vi "AlliGator Compute Shot Noise Average Lifetime Simulation Histograms.vi"(0 "Average Lifetimes (Pure Poisson)":dbl[](array[numeric]), 1 "Histogram Bin Size":dbl[unit], 5 "Average Lifetimes (AlliGator)":dbl[](array[numeric]), 7 "Lifetime Histo Percentiles":dbl[](array[numeric])=[99.0, 1.0], 9 "Average Lifetime SDVs (AlliGator)":dbl[](array[numeric]), 11 "Error In":errorcluster, 12 "Histogram Bin Size (SDV)":dbl[unit], 13 "SDV Histo Percentiles":dbl[](array[numeric])=[99.0, 1.0]) -> (3 "Histograms":cluster{"Axis":dbl[], "Histogram":dbl[]}[](array[cluster]), 4 "Array Statistic (Pure Poisson)":T1, 6 "Array Statistics (AlliGator)":T1, 10 "Array Statistics (AlliGator SDVs)":T1, 14 "Message":string, 15 "Error Out":errorcluster)   [LabVIEW 2021, in "AlliGator Shot Noise Influence on Average Lifetime.lvlib"]
doc: "Computes histograms and summary statistics for the computed lifetimes."
uses:
  AlliGator Shot Noise Influence on Average Lifetime.lvlib
  Arrays/Array Statistics.ctl
  Histograms/Linear Histogram Options.ctl
  Histograms/Histogram Bin Option.ctl
  Histograms/Histogram Bin Position.ctl
  5e0c3266-499e-46b2-80ef-c194e49f915b.vi
  9765538f-b151-4b8e-9b71-29b00fbc2fe4.vi
  8faa86fc-1a47-49e1-a18e-559db2184d30.vi
  c2a6bf4c-2b36-4ed5-885f-cf0e0406484b.vi
  6ac06ea2-d37e-43e0-baed-35fadc42c3ab.vi
  6045f332-e983-43bb-9ace-d0f5cff48457.vi
  5e0c3266-499e-46b2-80ef-c194e49f915b.vi/1ce800e1-bcd7-4855-83e2-66cab3687e54.vi
  9765538f-b151-4b8e-9b71-29b00fbc2fe4.vi/1ce800e1-bcd7-4855-83e2-66cab3687e54.vi
  8faa86fc-1a47-49e1-a18e-559db2184d30.vi/1ce800e1-bcd7-4855-83e2-66cab3687e54.vi
  c2a6bf4c-2b36-4ed5-885f-cf0e0406484b.vi/e021cd17-e000-4244-b7f4-ec50548bdfcb.vi
  c2a6bf4c-2b36-4ed5-885f-cf0e0406484b.vi/b1828c6e-eb0a-43e9-a724-8b596c52e435.vi
  c2a6bf4c-2b36-4ed5-885f-cf0e0406484b.vi/7a6138ed-c001-4311-b538-9ba42ae7c7b1.vi
  c2a6bf4c-2b36-4ed5-885f-cf0e0406484b.vi/52c6b4fa-501b-4af0-803b-8bab516ca5d3.vi
  c2a6bf4c-2b36-4ed5-885f-cf0e0406484b.vi/d7237e10-35ab-4bcb-a0c6-4883c3f4c990.vi
  c2a6bf4c-2b36-4ed5-885f-cf0e0406484b.vi/5fb5dd96-3b97-4592-ba56-58181c8e7105.vi
  c2a6bf4c-2b36-4ed5-885f-cf0e0406484b.vi/8e13a849-a393-4484-9968-4af7b25c38d7.vi
  6ac06ea2-d37e-43e0-baed-35fadc42c3ab.vi/e021cd17-e000-4244-b7f4-ec50548bdfcb.vi
  6ac06ea2-d37e-43e0-baed-35fadc42c3ab.vi/b1828c6e-eb0a-43e9-a724-8b596c52e435.vi
  6ac06ea2-d37e-43e0-baed-35fadc42c3ab.vi/7a6138ed-c001-4311-b538-9ba42ae7c7b1.vi
  6ac06ea2-d37e-43e0-baed-35fadc42c3ab.vi/52c6b4fa-501b-4af0-803b-8bab516ca5d3.vi
  6ac06ea2-d37e-43e0-baed-35fadc42c3ab.vi/d7237e10-35ab-4bcb-a0c6-4883c3f4c990.vi
  6ac06ea2-d37e-43e0-baed-35fadc42c3ab.vi/5fb5dd96-3b97-4592-ba56-58181c8e7105.vi
  6ac06ea2-d37e-43e0-baed-35fadc42c3ab.vi/8e13a849-a393-4484-9968-4af7b25c38d7.vi
  6045f332-e983-43bb-9ace-d0f5cff48457.vi/e021cd17-e000-4244-b7f4-ec50548bdfcb.vi
  6045f332-e983-43bb-9ace-d0f5cff48457.vi/b1828c6e-eb0a-43e9-a724-8b596c52e435.vi
  6045f332-e983-43bb-9ace-d0f5cff48457.vi/7a6138ed-c001-4311-b538-9ba42ae7c7b1.vi
  6045f332-e983-43bb-9ace-d0f5cff48457.vi/52c6b4fa-501b-4af0-803b-8bab516ca5d3.vi
  6045f332-e983-43bb-9ace-d0f5cff48457.vi/d7237e10-35ab-4bcb-a0c6-4883c3f4c990.vi
  6045f332-e983-43bb-9ace-d0f5cff48457.vi/5fb5dd96-3b97-4592-ba56-58181c8e7105.vi
  6045f332-e983-43bb-9ace-d0f5cff48457.vi/8e13a849-a393-4484-9968-4af7b25c38d7.vi
  Time/High Resolution Timing.vi
  <userlib>/_OpenG.lib/array/array.llb/Filter 1D Array__ogtk.vi
  <userlib>/_OpenG.lib/array/array.llb/Filter 1D Array (DBL)__ogtk.vi
  <userlib>/_OpenG.lib/array/array.llb/Delete Elements from Array__ogtk.vi
  <userlib>/_OpenG.lib/array/array.llb/Delete Elements from 1D Array (DBL)__ogtk.vi
  <vilib>/Utility/error.llb/Error Cluster From Error Code.vi
  Histograms/Histogram Window.lvlib
  Arrays/Arrays.lvlib
  Variant/Variant.lvlib
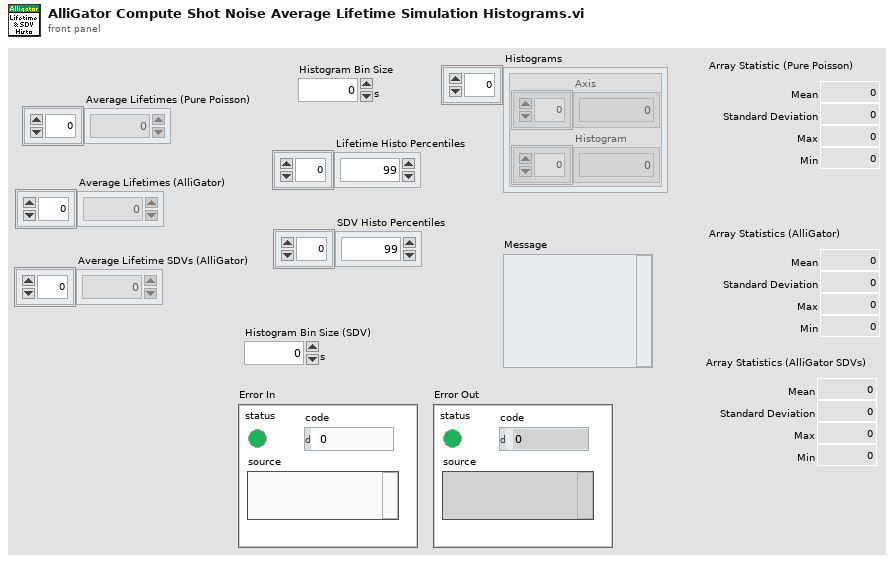
[diagram p1: front panel]
types:
  T1 = typedef "Arrays.lvlib/Array Statistics.ctl" = cluster{"Mean":dbl, "Standard Deviation":dbl, "Max":dbl, "Min":dbl}
  T2 = typedef "Histogram Window.lvlib/Linear Histogram Options.ctl" = cluster{"Bin Size":dbl, "Bin Number":i32, "Bin Option":T3, "Min Value":dbl, "Max Value":dbl, "Filter NaN & Infinite Values":bool, "Frequency Plot":bool, "Align Bins":bool, "Bin Location":T4, "Project Outside Values":bool, "Max Histogram Size":i32}
  T3 = typedef "Histogram Window.lvlib/Histogram Bin Option.ctl" = enum32{"Bin Number", "Bin Size"}
  T4 = typedef "Histogram Window.lvlib/Histogram Bin Position.ctl" = enum16{"Left", "Center", "Right"}
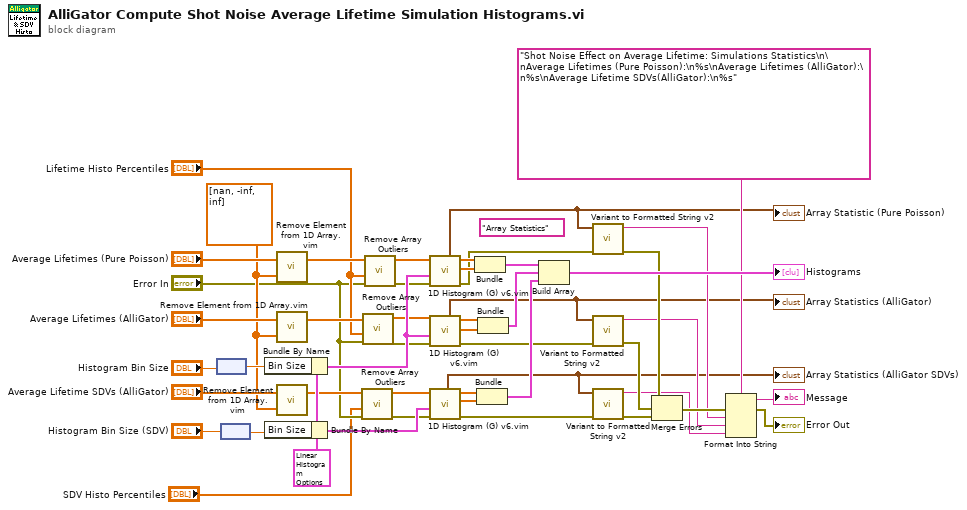
[diagram p0: block diagram]
diagram:
  (unwired) "Array Statistics" ("Label")
  w29 = dbl[] [nan, -inf, inf] ("Element(s) to Remove")
  w46 = T2 {"Bin Size"=nan, "Bin Number"=0, "Bin Option"=enum."Bin Size", "Min Value"=-inf, "Max Value"=inf, "Filter NaN & Infinite Values"=TRUE, "Frequency Plot"=FALSE, "Align Bins"=TRUE, "Bin Location"=enum."Left", "Project Outside Values"=FALSE, "Max Histogram Size"=100000} ("Histogram Options")
  n1 = node("Histogram Bin Size") -> (w42:dbl)
  n2 = node("Histogram Bin Size (SDV)") -> (w48:dbl)
  n3 = Bundle By Name(cluster=w46, "Bin Size"=w42) -> (w31:T2)
  n4 = Bundle By Name(cluster=w46, "Bin Size"=w48) -> (w49:T2)
  n5 = call "Remove Element from 1D Array.vim"("Element(s) to Remove"=w29, "Input Array"="Average Lifetimes (Pure Poisson)") -> ("Output Array"=w11:dbl[])  [unwired: 1 out]
  n6 = call "Remove Element from 1D Array.vim"("Element(s) to Remove"=w29, "Input Array"="Average Lifetimes (AlliGator)") -> ("Output Array"=w9:dbl[])  [unwired: 1 out]
  n7 = call "Remove Element from 1D Array.vim"("Element(s) to Remove"=w29, "Input Array"="Average Lifetime SDVs (AlliGator)") -> ("Output Array"=w6:dbl[])  [unwired: 1 out]
  n8 = call "Remove Array Outliers.vi"("Error In"="Error In", "Upper & Lower Percentile (100, 0)"="SDV Histo Percentiles", "Array in"=w6) -> ("Error Out"=w4:errorcluster, "Array out"=w5:dbl[])  [unwired: 6 in, 1 out]
  n9 = call "Remove Array Outliers.vi"("Error In"="Error In", "Upper & Lower Percentile (100, 0)"="Lifetime Histo Percentiles", "Array in"=w9) -> ("Error Out"=w7:errorcluster, "Array out"=w8:dbl[])  [unwired: 6 in, 1 out]
  n10 = call "Remove Array Outliers.vi"("Error In"="Error In", "Upper & Lower Percentile (100, 0)"="Lifetime Histo Percentiles", "Array in"=w11) -> ("Error Out"=w10:errorcluster, "Array out"=w12:dbl[])  [unwired: 6 in, 1 out]
  n11 = call "1D Histogram (G) v6.vim"("Error In"=w10, "Histogram Options"=w31, "Array"=w12) -> ("Error Out"=w25:errorcluster, "Histogram"=w33:dbl[], "Axis"=w32:dbl[], "Array Statistics"=w13:T1)  [unwired: 2 in, 3 out]
  "Array Statistic (Pure Poisson)" <- w13
  n12 = call "1D Histogram (G) v6.vim"("Error In"=w7, "Histogram Options"=w31, "Array"=w8) -> ("Error Out"=w24:errorcluster, "Histogram"=w35:dbl[], "Axis"=w34:dbl[], "Array Statistics"=w14:T1)  [unwired: 2 in, 3 out]
  "Array Statistics (AlliGator)" <- w14
  n13 = call "1D Histogram (G) v6.vim"("Error In"=w4, "Histogram Options"=w49, "Array"=w5) -> ("Error Out"=w23:errorcluster, "Histogram"=w37:dbl[], "Axis"=w36:dbl[], "Array Statistics"=w15:T1)  [unwired: 2 in, 3 out]
  "Array Statistics (AlliGator SDVs)" <- w15
  n14 = Bundle("Axis"=w32, "Histogram"=w33) -> (w38:cluster{"Axis":dbl[], "Histogram":dbl[]})  [unwired: 1 in]
  n15 = Bundle("Axis"=w36, "Histogram"=w37) -> (w40:cluster{"Axis":dbl[], "Histogram":dbl[]})  [unwired: 1 in]
  n16 = Bundle("Axis"=w34, "Histogram"=w35) -> (w39:cluster{"Axis":dbl[], "Histogram":dbl[]})  [unwired: 1 in]
  n17 = Build Array(w38, w39, w40) -> (→"Histograms":cluster{"Axis":dbl[], "Histogram":dbl[]}[])
  n18 = call "Variant to Formatted String v2.vi"("error in (no error)"=w25, "Anything"=w13) -> ("error out"=w22:errorcluster, "String"=w19:string)  [unwired: 8 in]
  n19 = call "Variant to Formatted String v2.vi"("error in (no error)"=w24, "Anything"=w14) -> ("error out"=w21:errorcluster, "String"=w18:string)  [unwired: 8 in]
  n20 = call "Variant to Formatted String v2.vi"("error in (no error)"=w23, "Anything"=w15) -> ("error out"=w20:errorcluster, "String"=w17:string)  [unwired: 8 in]
  n21 = Merge Errors(w22, w21, w20) -> (w28:errorcluster)
  n22 = Format Into String(format string="Shot Noise Effect on Average Lifetime: Simulations Statistics\n\nAverage Lifetimes (Pure Poisson):\n%s\nAverage Lifetimes (AlliGator):\n%s\nAverage Lifetime SDVs(AlliGator):\n%s", error in=w28, w19, w18, w17) -> (resulting string=→"Message":string, error out=→"Error Out":errorcluster)  [unwired: 1 in]
